vi "Encoder.vi"() -> (2 "Mes Pos (mm)":dbl[](array[numeric]), 3 "RPM":dbl[](array[knob]) scale=-200.0..200.0)   [LabVIEW 2021]
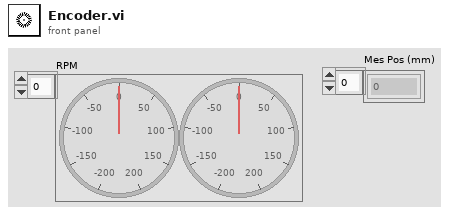
[diagram p1: front panel]
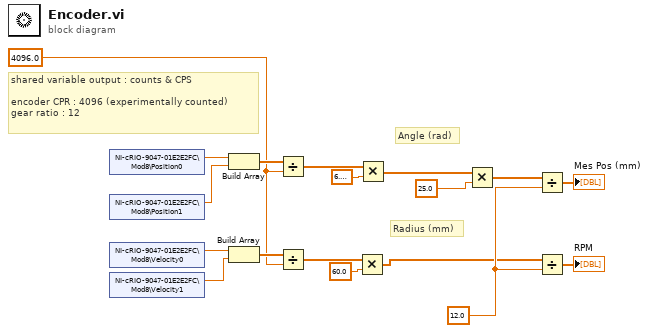
[diagram p0: block diagram]
diagram:
  w2 = 12.0 ("y")
  w7 = 4096.0 ("y")
  # "Radius (mm)"
  # "Angle (rad)"
  # "shared variable output : counts & CPS\n\nencoder CPR : 4096 (experimentally counted)\ngear ratio : 12"
  n1 = shared-variable "NI-cRIO-9047-01E2E2FC\\Mod8\\Position0"() -> (w12:dbl)  [unwired: 1 in, 1 out]
  n2 = shared-variable "NI-cRIO-9047-01E2E2FC\\Mod8\\Position1"() -> (w11:dbl)  [unwired: 1 in, 1 out]
  n3 = shared-variable "NI-cRIO-9047-01E2E2FC\\Mod8\\Velocity0"() -> (w16:dbl)  [unwired: 1 in, 1 out]
  n4 = shared-variable "NI-cRIO-9047-01E2E2FC\\Mod8\\Velocity1"() -> (w15:dbl)  [unwired: 1 in, 1 out]
  n5 = Build Array(w12, w11) -> (w13:dbl[])
  n6 = Build Array(w16, w15) -> (w14:dbl[])
  n7 = Divide(x=w13, y=w7) -> (x/y=w9:dbl[])
  n8 = Divide(x=w14, y=w7) -> (x/y=w18:dbl[])
  n9 = Multiply(x=w18, y=60.0) -> (x*y=w1:dbl[])
  n10 = Multiply(x=w9, y=6.283185307179586) -> (x*y=w6:dbl[])
  n11 = Multiply(x=w6, y=25.0) -> (x*y=w4:dbl[])
  n12 = Divide(x=w4, y=w2) -> (x/y=→"Mes Pos (mm)":dbl[])
  n13 = Divide(x=w1, y=w2) -> (x/y=→"RPM":dbl[])
